vi "Set_Tab_Num_Relay.vi"(8 "error in (no error)":errorcluster caption="entrée d'erreur (pas d'erreur)", 10 "Tab_Num_Relay":u8[](array[numeric]), 11 "Instrument Relay_Board en entrée":refnum<class "Class Instrument Relay_Board.lvclass">) -> (0 "error out":errorcluster caption="sortie d'erreur", 3 "Instrument Relay_Board en sortie":refnum<class "Class Instrument Relay_Board.lvclass">)   [LabVIEW 2020, in "Library Instrument & Equipement.lvlib" / "Library Instruments.lvlib" / "Class Instrument Relay_Board.lvclass"]
uses:
  Class Instrument Relay_Board.lvclass
  Class Instrument Relay_Board.lvclass/Class Instrument Relay_Board.ctl
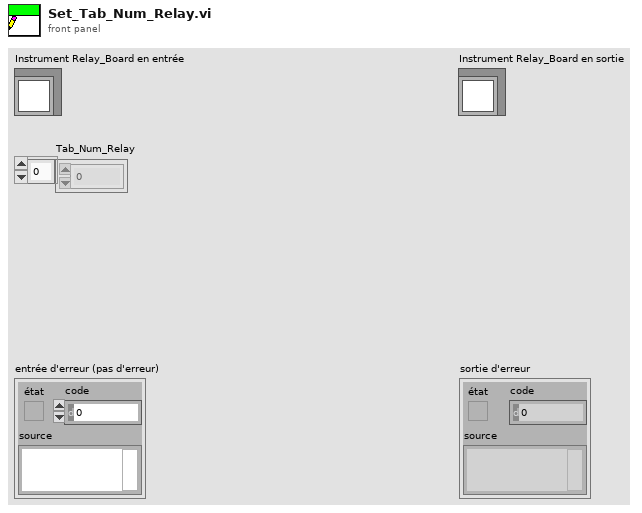
[diagram p1: front panel]
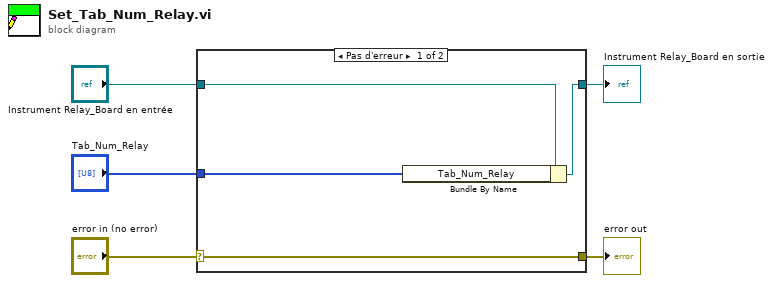
[diagram p0: block diagram]
diagram:
  n1 = case shown="Pas d'erreur" "error in (no error)" {
    selector: "error in (no error)" -> [w9 w10]
    tunnel: [w9 w10] -> w4
    tunnel: [w7 w11] -> w2
    tunnel: "Instrument Relay_Board en entrée" -> [w8 w11]
    tunnel: "Tab_Num_Relay" -> [w6 _]
    frame No Error {
      n2 = Bundle By Name(cluster=w8, "Tab_Num_Relay"=w6) -> (w7:refnum<class "Class Instrument Relay_Board.lvclass">)
    }
    frame Error {
    }
  }
  "error out" <- w4
  "Instrument Relay_Board en sortie" <- w2
